vi "countResults.vi"(11 "TopResultList":refnum<k7>) -> (3 "Results Qtys":T1)   [LabVIEW 2025]
uses:
  <vilib>/Utility/error.llb/Trim Whitespace One-Sided.vi
panel:
  # "To be called in Main cleanup callback; \npass in object: Locals.ResultList"
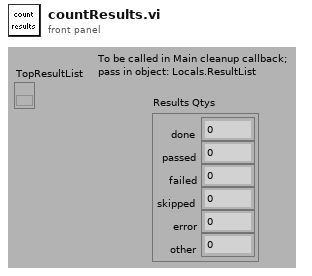
[diagram p1: front panel]
types:
  T1 = cluster{"done":i32, "passed":i32, "failed":i32, "skipped":i32, "error":i32, "other":i32}
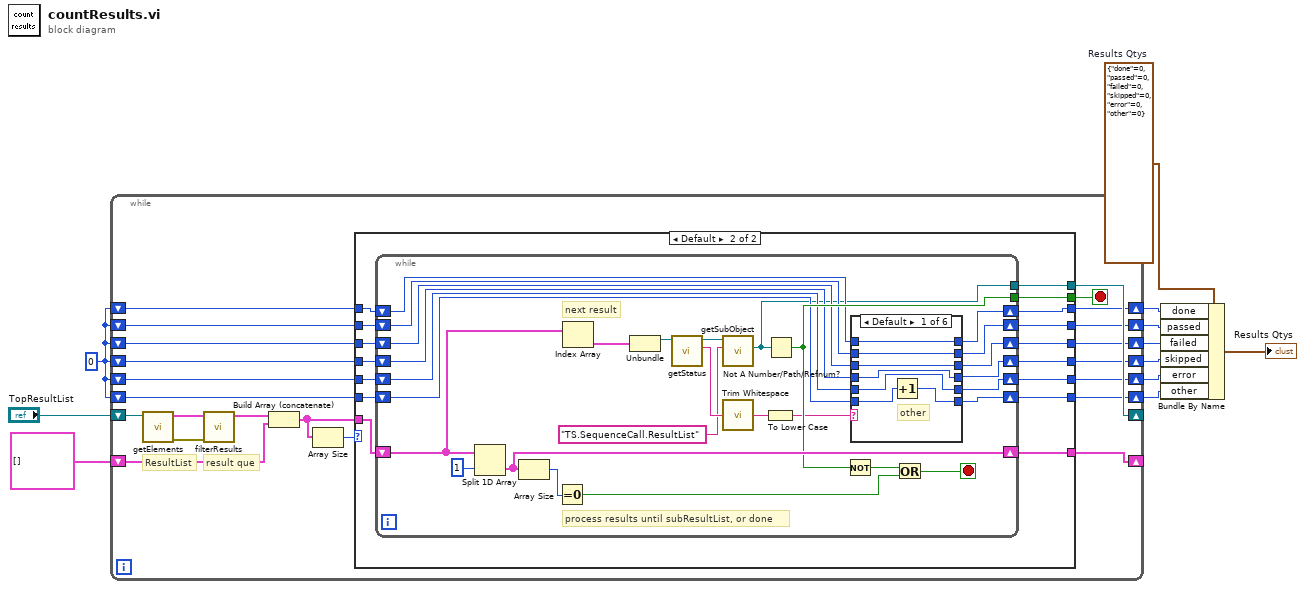
[diagram p0: block diagram]
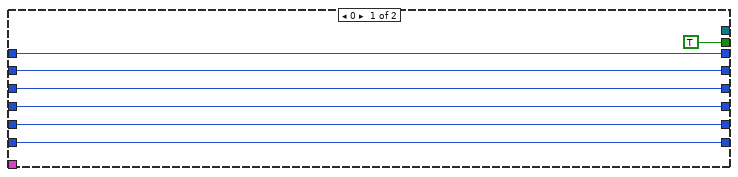
[diagram p2: hidden frame]
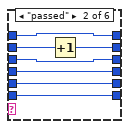
[diagram p3: hidden frame]
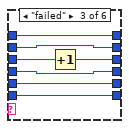
[diagram p4: hidden frame]
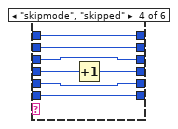
[diagram p5: hidden frame]
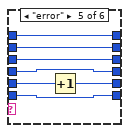
[diagram p6: hidden frame]
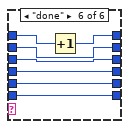
[diagram p7: hidden frame]
diagram:
  w2 = 0
  w9 = T1 {"done"=0, "passed"=0, "failed"=0, "skipped"=0, "error"=0, "other"=0}  # Results Qtys
  n1 = while {
    shift-right: [w30] -> _
    shift-left: cluster{"Object":refnum<k7>, "level":i32}[] [] -> [w29]
    shift-right: [w31] -> _
    shift-left: "TopResultList" -> [w33]
    shift-right: [w23] -> w7
    shift-left: w2 -> [w22]
    shift-right: [w20] -> w6
    shift-left: w2 -> [w21]
    shift-right: [w19] -> w4
    shift-left: w2 -> [w18]
    shift-right: [w16] -> w5
    shift-left: w2 -> [w17]
    shift-right: [w14] -> w3
    shift-left: w2 -> [w15]
    shift-right: [w12] -> w1
    shift-left: w2 -> [w13]
    stop <- w26 stop-if-true
    # "ResultList"
    # "result que"
    n2 = call "getElements.vi"("resultList"=w33) -> ("error out"=w27:errorcluster, "elements"=w32:cluster{"Object":refnum<k7>, i32}[])  [unwired: 2 in, 7 out]
    n3 = call "filterResults.vi"("error in"=w27, "Array in"=w32) -> ("Array"=w28:cluster{"Object":refnum<k7>, i32}[])  [unwired: 1 in, 8 out]
    n4 = Build Array (concatenate)(w28, w29) -> (w25:cluster{"Object":refnum<k7>, "level":i32}[])
    n5 = Array Size(array=w25) -> (size(s)=w24:i32)
    n6 = case shown="Default" w24 {
      tunnel: [_ w56] -> w31
      tunnel: [_ w55] -> w30
      tunnel: w25 -> [_ w54]
      tunnel: [TRUE w53] -> w26
      tunnel: [w39 w52] -> w23
      tunnel: w22 -> [w39 w45]
      tunnel: w21 -> [w34 w41]
      tunnel: [w34 w51] -> w20
      tunnel: [w37 w50] -> w19
      tunnel: w18 -> [w37 w44]
      tunnel: w17 -> [w36 w43]
      tunnel: [w36 w49] -> w16
      tunnel: w15 -> [w35 w42]
      tunnel: [w35 w48] -> w14
      tunnel: w13 -> [w38 w46]
      tunnel: [w38 w47] -> w12
      frame 0 {
      }
      frame Default {
        n7 = while {
          tunnel: [w57] -> w56
          shift-right: [w82] -> w55
          shift-left: w54 -> [w84]
          tunnel: [w77] -> w53
          shift-right: [w71] -> w47
          shift-left: w46 -> [w70]
          shift-right: [w76] -> w52
          shift-left: w45 -> [w69]
          shift-right: [w74] -> w50
          shift-left: w44 -> [w68]
          shift-right: [w73] -> w49
          shift-left: w43 -> [w67]
          shift-right: [w72] -> w48
          shift-left: w42 -> [w66]
          shift-right: [w75] -> w51
          shift-left: w41 -> [w65]
          stop <- w78 stop-if-true
          # "next result"
          # "process results until subResultList, or done"
          n8 = Split 1D Array(array=w84, index=1) -> (second subarray=w82:cluster{"Object":refnum<k7>, "level":i32}[])  [unwired: 1 out]
          n9 = Array Size(array=w82) -> (size(s)=w83:i32)
          n10 = Equal To 0?(x=w83) -> (x = 0?=w80:bool)
          n11 = Index Array(array=w84) -> (element=w62:cluster{"Object":refnum<k7>, "level":i32})  [unwired: 1 in]
          n12 = Unbundle(w62) -> ("Object"=w61:refnum<k7>)  [unwired: 1 out]
          n13 = call "getStatus.vi"("Object"=w61) -> ("string"=w60:string, "Object Out"=w59:refnum<k7>)  [unwired: 1 in, 8 out]
          n14 = call "getSubObject.vi"("lookup"="TS.SequenceCall.ResultList", "parent"=w59) -> ("subobject"=w57:refnum<k7>)  [unwired: 1 in, 8 out]
          n15 = call <vilib>:"Trim Whitespace.vi"("string"=w60) -> ("trimmed string"=w63:string)  [unwired: 1 in]
          n16 = To Lower Case(string=w63) -> (all lower case string=w64:string)
          n17 = Not A Number/Path/Refnum?(number/path/refnum=w57) -> (NaN/Path/Refnum?=w77:bool)
          n18 = Not(x=w77) -> (.not. x?=w79:bool)
          n19 = case shown="Default" w64 {
            tunnel: [w91 w98 w102 w111 w118 w125] -> w76
            tunnel: w69 -> [w91 w97 w102 w111 w118 w125]
            tunnel: w65 -> [w90 w96 w105 w112 w119 w126]
            tunnel: [w89 w96 w105 w112 w119 w126] -> w75
            tunnel: [w88 w95 w104 w110 w117 w124] -> w74
            tunnel: w68 -> [w88 w95 w103 w110 w117 w124]
            tunnel: w67 -> [w87 w94 w101 w109 w116 w123]
            tunnel: [w87 w94 w101 w108 w116 w123] -> w73
            tunnel: w66 -> [w86 w93 w100 w107 w115 w122]
            tunnel: [w86 w93 w100 w107 w114 w122] -> w72
            tunnel: w70 -> [w85 w92 w99 w106 w113 w121]
            tunnel: [w85 w92 w99 w106 w113 w120] -> w71
            frame Default {
              # "other"
              n20 = Increment(x=w90) -> (x+1=w89:i32)
            }
            frame "passed" {
              n21 = Increment(x=w97) -> (x+1=w98:i32)
            }
            frame "failed" {
              n22 = Increment(x=w103) -> (x+1=w104:i32)
            }
            frame "skipmode", "skipped" {
              n23 = Increment(x=w109) -> (x+1=w108:i32)
            }
            frame "error" {
              n24 = Increment(x=w115) -> (x+1=w114:i32)
            }
            frame "done" {
              n25 = Increment(x=w121) -> (x+1=w120:i32)
            }
          }
          n26 = Or(x=w79, y=w80) -> (x .or. y?=w78:bool)
        }
      }
    }
  }
  n27 = Bundle By Name(cluster=w9, "done"=w1, "passed"=w7, "failed"=w4, "skipped"=w5, "error"=w3, "other"=w6) -> (→"Results Qtys":T1)
